vi "Write Report.vi"(8 "error in (no error)":errorcluster, 10 "Resource In":variant, 11 "Width Method in":refnum<class "Width Method.lvclass">) -> (0 "error out":errorcluster, 2 "Resource Out":variant, 3 "Width Method out":refnum<class "Width Method.lvclass">)   [LabVIEW 2020, in "Width Method.lvclass"]
uses:
  Width Method.lvclass
  C:/POLARIS Programme/POLARIS-AS-3-Cams/Submodules/HIJ Vision/Analyze/Analyze Parameter/Analyze Parameter Base/Analyze Parameter Base.lvclass
  Analyze Classes/Width Method.ctl
  <vilib>/Utility/config.llb/Config Data RefNum.ctl
  Width Method.lvclass/Width Method.ctl
  <vilib>/Utility/config.llb/Write Key (String).vi
  <vilib>/Utility/config.llb/NI_LVConfig.lvlib
  Analyze Classes/Analyze.lvlib
panel:
  out "Width in":T1
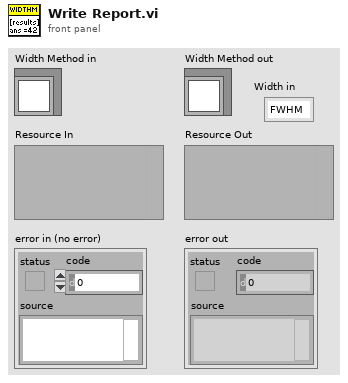
[diagram p1: front panel]
types:
  T1 = typedef "Analyze.lvlib/Width Method.ctl" = enum16{"FWHM", "1/e", "1/e^2", "80%", "90%"}
  T2 = typedef "NI_LVConfig.lvlib/Config Data RefNum.ctl" = refnum<k1>
  T3 = typedef "POLARIS Vision utility.lvlib/Width Method.ctl" = enum16{"FWHM", "1/e", "1/e^2", "80%", "90%"}
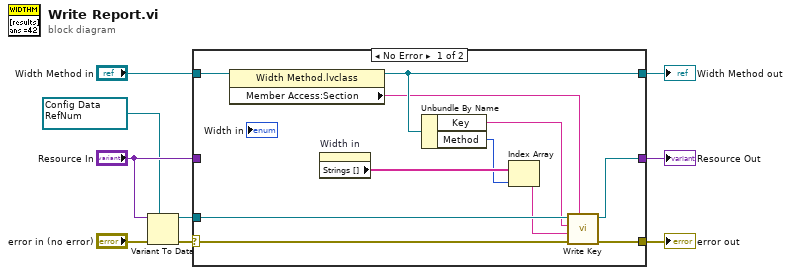
[diagram p0: block diagram]
diagram:
  w7 = T2 refnum items=["config data"] ("refnum")
  n1 = Variant To Data(error in="error in (no error)", type=w7, Variant="Resource In") -> (data=w8:T2, error out=w1:errorcluster)
  n2 = case shown="No Error" w1 {
    selector: w1 -> [w14 w22]
    tunnel: w8 -> [w20 _]
    tunnel: "Width Method in" -> [w19 w21]
    tunnel: [w18 w21] -> w5
    tunnel: [w15 w23] -> w4
    tunnel: [w16 w22] -> w3
    tunnel: "Resource In" -> [_ w23]
    frame No Error {
      n3 = property class="Width Method.lvclass"(reference=w19) -> (reference out=w18:refnum<class "Width Method.lvclass">, "Member Access:Section"=w17:string)  [unwired: 1 in, 1 out]
      n4 = property on="Width in" class="Enum (strict)"() -> ("Strings []"=w12:string[])  [unwired: 2 in, 2 out]
      n5 = Unbundle By Name(w18) -> ("Key"=w13:string, "Method"=w11:T3)
      n6 = Index Array(array=w12, index=w11) -> (element=w10:string)
      n7 = call-poly <vilib>:"Write Key.vi"("section"=w17, "error in (no error)"=w14, "value"=w10, "key"=w13, "refnum"=w20) -> ("error out"=w16:errorcluster, "refnum out"=w15:T2)  [unwired: 4 in, 1 out]
    }
    frame Error {
    }
  }
  "error out" <- w3
  "Width Method out" <- w5
  "Resource Out" <- w4
